vi "CDMA_RxSCSearch.vi"(7 "scrambleGroupNo":dbl, 8 "error in (no error)":errorcluster caption="错误输入（无错误）", 9 "sampleRate":dbl, 10 "rx_data1":cdb[](array[numeric]), 11 "Path In":path) -> (0 "error out":errorcluster caption="错误输出", 1 "scramblingCode":cdb[](array[numeric]), 2 "scrambleNo":dbl, 3 "Path Out":path)   [LabVIEW 2015]
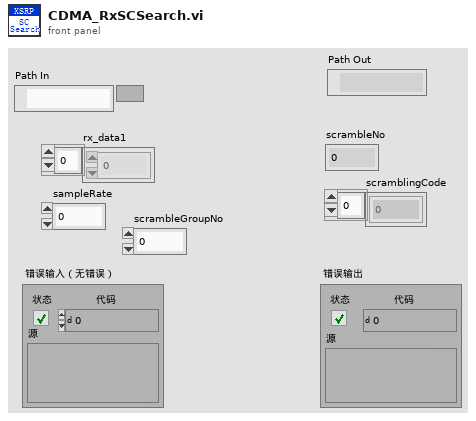
[diagram p1: front panel]
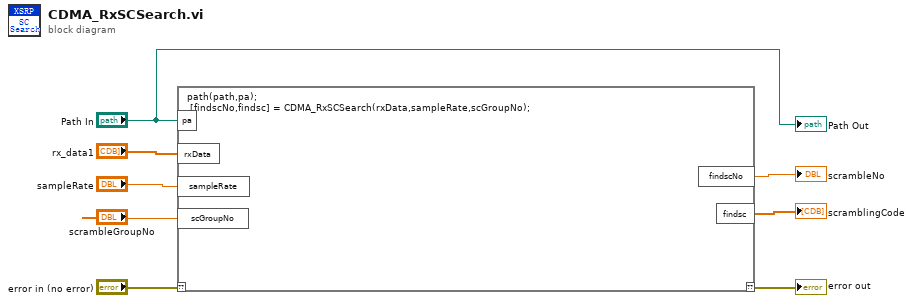
[diagram p0: block diagram]
diagram:
  n1 = script code="path(path,pa);\n [findscNo,findsc] = CDMA_RxSCSearch(rxData,sampleRate,scGroupNo);"("??"="error in (no error)", "pa"="Path In", "rxData"="rx_data1", "sampleRate"="sampleRate", "scGroupNo"="scrambleGroupNo") -> ("??"=→"error out":errorcluster, "findscNo"=→"scrambleNo":dbl, "findsc"=→"scramblingCode":cdb[])
  "Path Out" <- "Path In"
